vi "Hanning Filter Extended.vi"(7 "Control":enum16{"Init", "Filter"}(ring), 10 "Input 2":dbl, 11 "Input":dbl) -> (2 "Filtered2":dbl, 3 "Filtered":dbl)   [LabVIEW 2013]
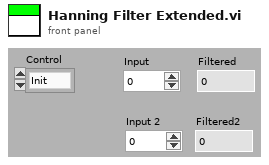
[diagram p1: front panel]
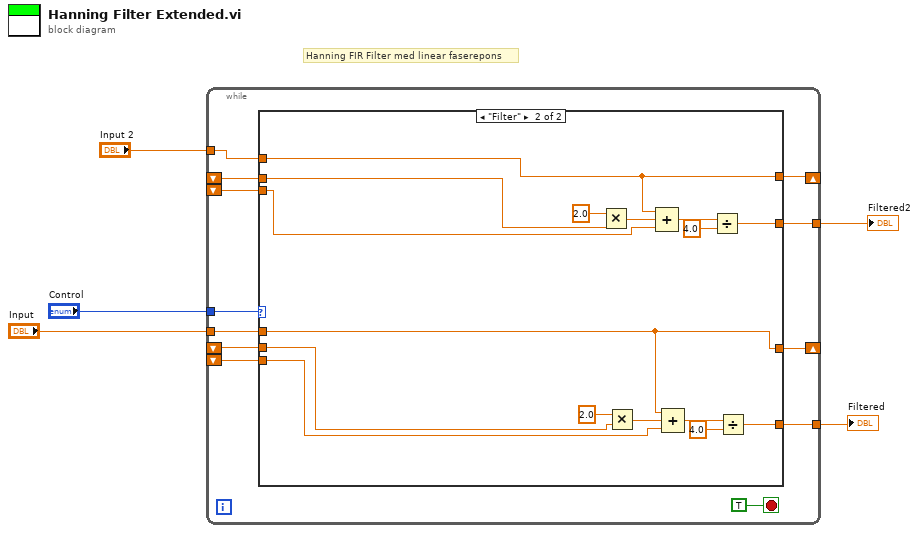
[diagram p0: block diagram]
diagram:
  # "Hanning FIR Filter med linear faserepons"
  n1 = while {
    shift-right: [w17] -> _
    shift-left: _ -> [w16]
    tunnel: "Input" -> [w15]
    tunnel: "Control" -> [w14]
    tunnel: [w12] -> w3
    shift-left: _ -> [w11]
    shift-right: [w9] -> _
    shift-left: _ -> [w8]
    tunnel: "Input 2" -> [w10]
    shift-left: _ -> [w7]
    tunnel: [w6] -> w1
    stop <- TRUE stop-if-true
    n2 = case shown="\"Filter\"" w14 {
      tunnel: [w18 w20] -> w17
      tunnel: w16 -> [_ w22]
      tunnel: w15 -> [w18 w20]
      tunnel: [w18 w31] -> w12
      tunnel: w11 -> [_ w21]
      tunnel: [w19 w25] -> w9
      tunnel: w10 -> [w19 w25]
      tunnel: w8 -> [_ w24]
      tunnel: w7 -> [_ w23]
      tunnel: [w19 w26] -> w6
      frame "Init" {
      }
      frame "Filter" {
        n3 = Multiply(x=2.0, y=w24) -> (x*y=w29:dbl)
        n4 = Multiply(x=2.0, y=w22) -> (x*y=w34:dbl)
        n5 = Compound Arithmetic op=ADD(w25, w29, w23) -> (w28:dbl)
        n6 = Compound Arithmetic op=ADD(w20, w34, w21) -> (w33:dbl)
        n7 = Divide(x=w28, y=4.0) -> (x/y=w26:dbl)
        n8 = Divide(x=w33, y=4.0) -> (x/y=w31:dbl)
      }
    }
  }
  "Filtered" <- w3
  "Filtered2" <- w1
